vi "Ejercicio_9_Filtro_EMA.vi"(10 "stop":bool, 11 "Array":dbl[](array[numeric])) -> (2 "appended array 2":dbl[](array[numeric]), 3 "appended array":dbl[](array[numeric]))   [LabVIEW 2020]
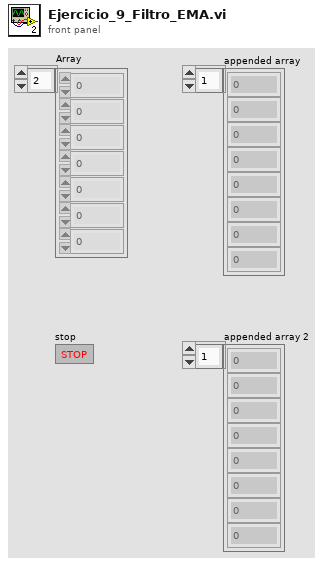
[diagram p1: front panel]
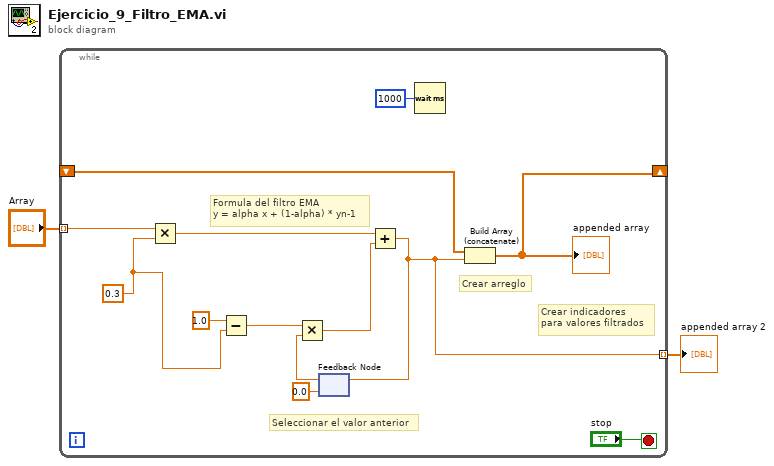
[diagram p0: block diagram]
diagram:
  n1 = while {
    tunnel: "Array" -> [w13] mode=indexing
    shift-right: [w5] -> _
    shift-left: _ -> [w4]
    tunnel: [w3] -> w2 mode=indexing
    stop <- "stop" stop-if-true
    w10 = 0.3 ("y")
    # "Crear indicadores \npara valores filtrados"
    # "Crear arreglo"
    # "Formula del filtro EMA\ny = alpha x + (1-alpha) * yn-1"
    # "Seleccionar el valor anterior"
    n2 = Multiply(x=w13, y=w10) -> (x*y=w12:dbl)
    n3 = Subtract(x=1.0, y=w10) -> (x-y=w9:dbl)
    n4 = feedback #1(0.0) -> (w7:dbl)
    n5 = Multiply(x=w9, y=w7) -> (x*y=w8:dbl)
    n6 = Add(x=w12, y=w8) -> (x+y=w3:dbl)
    n7 = feedback-in #1(w3) -> ()
    n8 = Wait (ms)(milliseconds to wait=u32 1000) -> ()  [unwired: 1 out]
    n9 = Build Array (concatenate)(w4, w3) -> (w5:dbl[])
    "appended array" <- w5
  }
  "appended array 2" <- w2
